vi "COBS_Stuff.vi"(8 "error in (no error)":errorcluster, 11 "Raw data":string) -> (0 "error out":errorcluster, 3 "Stuffed Data":string)   [LabVIEW 2015, in "Shore Library.lvlib"]
doc: "Stuffs a u8 array with the COBS algorithm. This is used to take zeros out of a byte array to allow it to be used as a delimeter. \n\nhttps://en.wikipedia.org/wiki/Consistent_Overhead_Byte_Stuffing"
uses:
  Shore Library.lvlib
panel:
  out "Array out":u8[](array[numeric])
  in  "Array in":u8[](array[numeric])
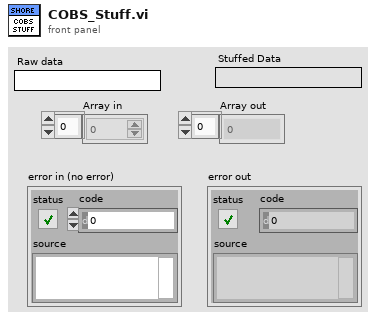
[diagram p1: front panel]
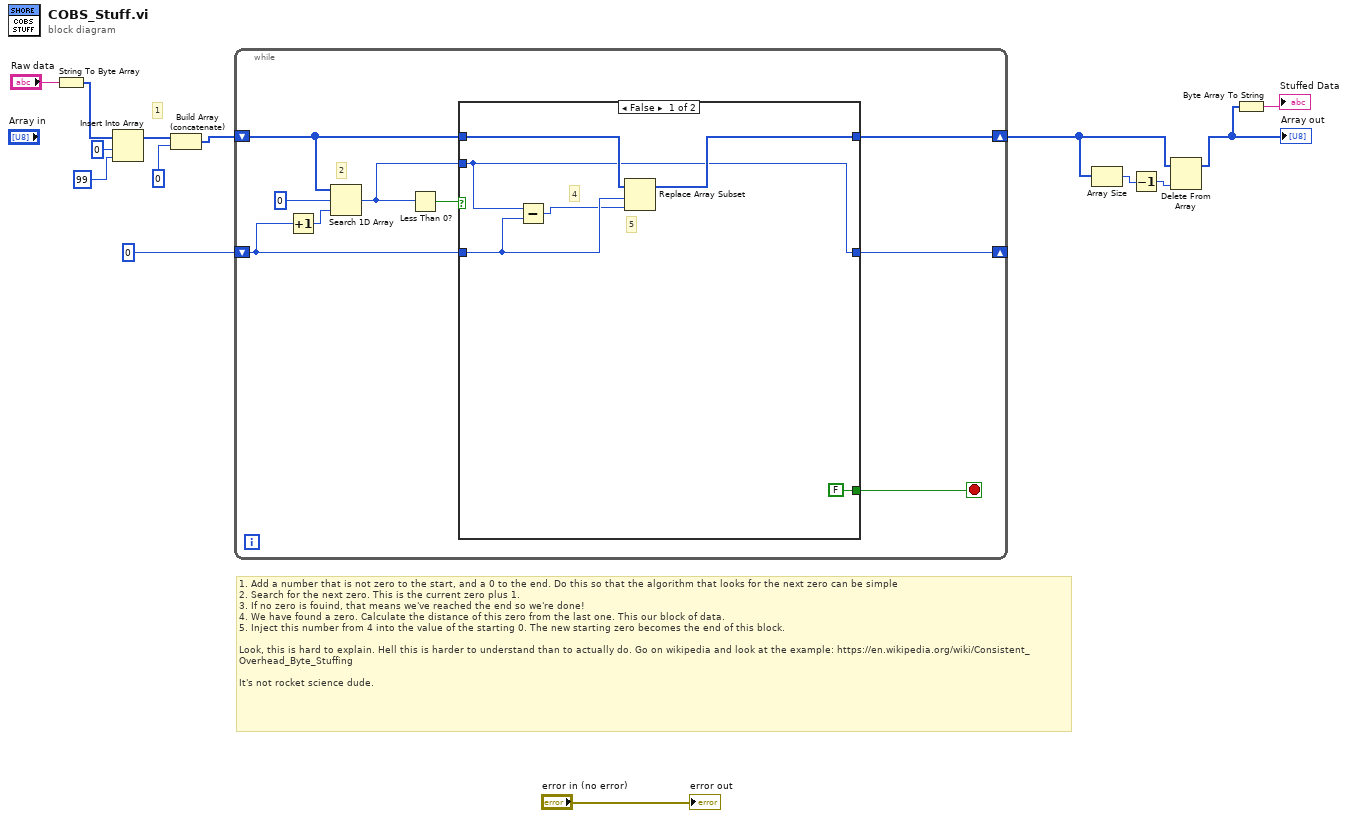
[diagram p0: block diagram]
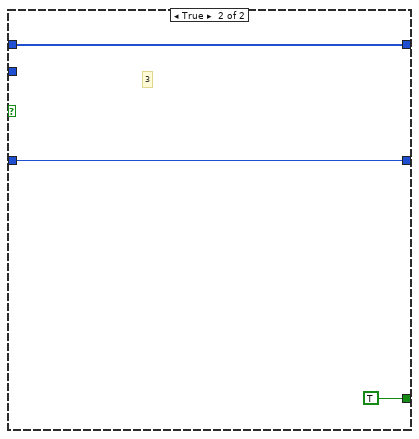
[diagram p2: hidden frame]
diagram:
  # "1. Add a number that is not zero to the start, and a 0 to the end. Do this so that the algorithm that looks for the next zero can be simple\n2. Search for the next zero. This is the current zero plus 1. \n3. If no zero is fouind, that means we've reached the end so we're done!\n4. We have found a zero. Calculate the distance of this zero from the last one. This our block of data.\n5. Inject this number from 4 into the value of the starting 0. The new starting zero becomes the end of this block.\n\nLook, this is hard to explain. Hell this is harder to understand than to actually do. Go on wikipedia and look at the example: https://en.wikipedia.org/wiki/Consistent_Overhead_Byte_Stuffing\n\nIt's not rocket science dude."
  # "1"
  n1 = String To Byte Array(string="Raw data") -> (unsigned byte array=w1:u8[])
  n2 = Insert Into Array(array=w1, index=0, new element=u8 99 ("element")) -> (w12:u8[])
  n3 = Build Array (concatenate)(w12, u8 0 ("element")) -> (w13:u8[])
  n4 = while {
    shift-right: [w15] -> w5
    shift-left: w13 -> [w22]
    shift-right: [w19] -> _
    shift-left: u8 0 ("element") -> [w16]
    stop <- w21 stop-if-true
    # "2"
    n5 = Increment(x=w16) -> (x+1=w17:i32)
    n6 = Search 1D Array(1D array=w22, element=u8 0, start index (0)=w17) -> (index of element=w18:i32)
    n7 = Less Than 0?(x=w18) -> (x < 0?=w20:bool)
    n8 = case shown="False" w20 {
      tunnel: [w25 w30] -> w15
      tunnel: w22 -> [w26 w30]
      tunnel: [FALSE TRUE] -> w21
      tunnel: w16 -> [w28 w31]
      tunnel: [w24 w31] -> w19
      tunnel: w18 -> [w24 _]
      frame False {
        # "5"
        # "4"
        n9 = Subtract(x=w24, y=w28) -> (x-y=w27:i32)
        n10 = Replace Array Subset(array=w26, new element=w27, index=w28) -> (w25:u8[])
      }
      frame True {
        # "3"
      }
    }
  }
  n11 = Array Size(array=w5) -> (size(s)=w7:i32)
  n12 = Decrement(x=w7) -> (x-1=w6:i32)
  n13 = Delete From Array(array=w5, index=w6) -> (array with subset deleted=w3:u8[])  [unwired: 1 in, 1 out]
  "Array out" <- w3
  n14 = Byte Array To String(unsigned byte array=w3) -> (string=→"Stuffed Data":string)
  "error out" <- "error in (no error)"
